vi "SwissSPAD Live_Process Displayed Image.vi"(8 "Error In":errorcluster, 11 "Refnum in":T1) -> (0 "Error Out":errorcluster, 3 "Refnum out":T1)   [LabVIEW 2021]
uses:
  <vilib>/vision/Image Controls.llb/IMAQ Image.ctl
  SwissSPAD Live_Settings List.ctl
  SwissSPAD Live_Image Display Options.ctl
  SwissSPAD Live_Internal Data List.ctl
  Variant/Variant to Data/Variant to Data.lvlib
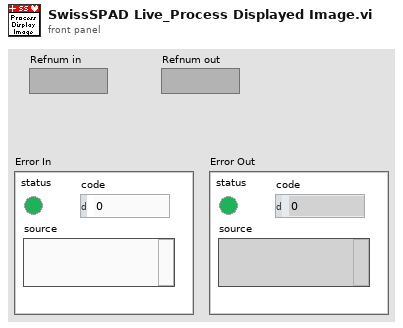
[diagram p1: front panel]
types:
  T1 = typedef "IMAQ Image.ctl" = refnum<image>
  T2 = typedef "SwissSPAD Live_Internal Data List.ctl" = enum16{"Number of pending file saving tasks", "File Saving Tasks Information", "Current Image ROI Information", "# FPGA Reset Attempts", "Histogram Cursor Locations", "Histogram Window is Open"}
  T3 = typedef "SwissSPAD Live_Settings List.ctl" = enum16{"FPGA:Bottom Half", "FPGA:Top Half", "FPGA:Bottom Bitfile Path", "FPGA:Top Bitfile Path", "FPGA:Bottom Bitstream Version", "FPGA:Top Bitstream Version", "FPGA:Auto Reset FPGA", "FPGA:Bottom FPGA Serial Number", "FPGA:Top FPGA Serial Number", "FPGA:Detector PCB Version", "Acquisition Parameters:Microlens", "Acquisition Parameters:SS2 DAQ Parameters", "Acquisition Parameters:Gate Configuration Array", "Acquisition Parameters:SS3 DAQ Parameters", "Acquisition Parameters:Buffer Size (# 8-bit Gates)", "File Information:File Information", "File Information:# Datasets in Series", "File Information:Scrambled File Flag", "File Information:SS3 Gate Slip Correction", "File Information:SS3 Hot Pixel Mismatch Detection", "File Information:Delay between Datasets", "File Information:Save Sum of All Gates Preview", "Image Parameters:Image ROI Information", "Image Parameters:Image Binning Options", "Image Parameters:SS3 Displayed Image", "Image Parameters:Image Display Options", "Image Parameters:Use Histogram Cursors", "Image Parameter:FPGA Data to Display", "UI Settings:Histogram Bins Number", "UI Settings:Histogram Bin Size", "UI Settings:Use Image Display Options", "UI Settings:Verbose Settings", "UI Settings:Verbose Saving"}
  T4 = typedef "SwissSPAD Live_Image Display Options.ctl" = cluster{"Remove Screamers":bool, "Delta":sgl, "Equalize Histogram":bool, "Percentile":sgl, "Hot Pixel Mask Image":path, "Use Hot Pixel Mask":bool}
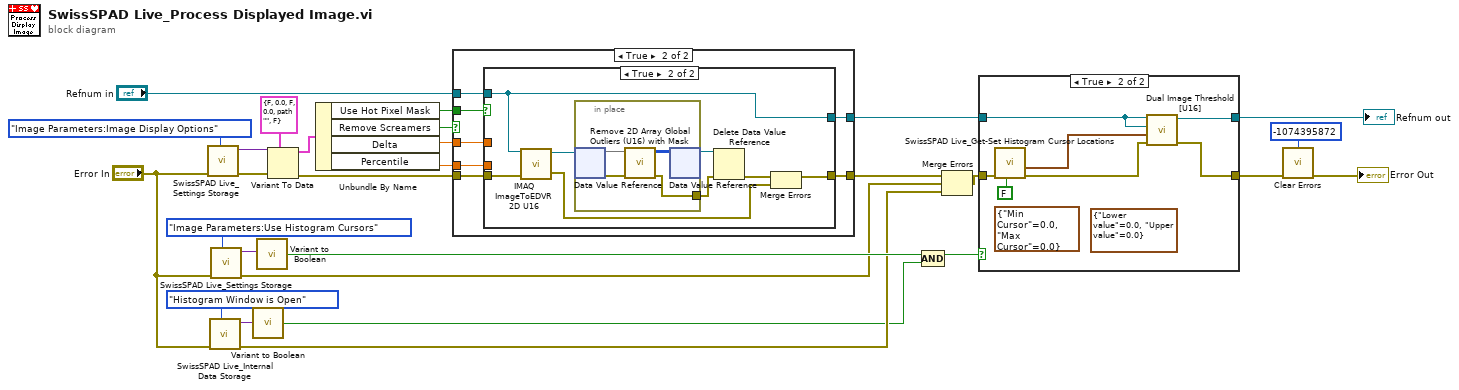
[diagram p0: block diagram]
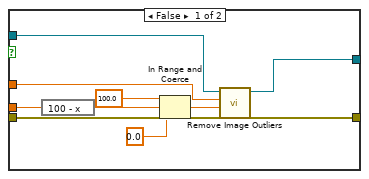
[diagram p4: hidden frame]
diagram:
  n1 = call "SwissSPAD Live_Settings Storage.vi"("Settings List"=SwissSPAD_Live_Settings_List."Image Parameters:Image Display Options", "Error In"="Error In") -> ("Error Out"=w28:errorcluster, "Variant Data out"=w10:variant)  [unwired: 8 in]
  n2 = call "SwissSPAD Live_Internal Data Storage.vi"("SS2 Live Data"=SwissSPAD_Live_Internal_Data_List."Histogram Window is Open", "Error In"="Error In") -> ("Error Out"=w4:errorcluster, "Variant"=w3:variant)  [unwired: 7 in, 1 out]
  n3 = call "SwissSPAD Live_Settings Storage.vi"("Settings List"=SwissSPAD_Live_Settings_List."Image Parameters:Use Histogram Cursors", "Error In"="Error In") -> ("Error Out"=w5:errorcluster, "Variant Data out"=w11:variant)  [unwired: 8 in]
  n4 = call "Variant to Boolean.vi"("Variant"=w3) -> ("Value"=w1:bool)  [unwired: 8 in]
  n5 = call "Variant to Boolean.vi"("Variant"=w11) -> ("Value"=w18:bool)  [unwired: 8 in]
  n6 = Variant To Data(error in=w28, type=T4 {"Remove Screamers"=FALSE, "Delta"=0.0, "Equalize Histogram"=FALSE, "Percentile"=0.0, "Hot Pixel Mask Image"=path "", "Use Hot Pixel Mask"=FALSE} ("Image Display Options"), Variant=w10) -> (data=w26:T4, error out=w25:errorcluster)
  n7 = Unbundle By Name(w26) -> ("Use Hot Pixel Mask"=w9:bool, "Remove Screamers"=w23:bool, "Delta"=w24:sgl, "Percentile"=w21:sgl)
  n8 = case shown="True" w23 {
    tunnel: w25 -> [w29 w37]
    tunnel: w24 -> [_ w36]
    tunnel: [w29 w35] -> w17
    tunnel: "Refnum in" -> [w30 w34]
    tunnel: [w30 w33] -> w16
    tunnel: w21 -> [_ w32]
    tunnel: w9 -> [_ w31]
    frame False {
    }
    frame True {
      n9 = case shown="True" w31 {
        tunnel: w37 -> [w47 w55]
        tunnel: w36 -> [w46 _]
        tunnel: [w45 w49] -> w35
        tunnel: w34 -> [w44 w50]
        tunnel: [w43 w50] -> w33
        tunnel: w32 -> [w42 _]
        frame False {
          n10 = expression code="100 - x"(w42) -> (w41:sgl)
          n11 = In Range and Coerce(upper limit=sgl 100.0, x=w41, lower limit=sgl 0.0) -> (coerced(x)=w40:sgl)  [unwired: 1 out]
          n12 = call "Remove Image Outliers.vi"("error in (no error)"=w47, "Percentile (0-100, Default: ignore)"=w40, "Delta (Default: ignore)"=w46, "Refnum in"=w44) -> ("error out"=w45:errorcluster, "Refnum out"=w43:T1)  [unwired: 6 in]
        }
        frame True {
          n13 = call <vilib>:"IMAQ ImageToEDVR 2D U16.vi"("error out"=w55, "Image"=w50) -> ("error out"=w48:errorcluster, "EDVR 2D U16"=w54:refnum<data-value>)  [unwired: 7 in, 1 out]
          n14 = in-place {
            in-place-border: [w56] -> w52
            n15 = in-place-dvr #1(w54) -> (w59:u16[][], w58:errorcluster)
            n16 = call "Remove 2D Array Global Outliers (U16) with Mask.vi"("Error In"=w58, "2D Array in"=w59) -> ("Error Out"=w56:errorcluster, "2D Array out"=w57:u16[][])  [unwired: 6 in, 2 out]
            n17 = in-place-dvr #1(w57) -> (w53:refnum<data-value>)  [unwired: 1 out]
          }
          n18 = Delete Data Value Reference(data value reference=w53, error in=w52) -> (error out=w51:errorcluster)  [unwired: 1 out]
          n19 = Merge Errors(w51, w48) -> (w49:errorcluster)
        }
      }
    }
  }
  n20 = Compound Arithmetic op=AND(w18, w1) -> (w2:bool)
  n21 = Merge Errors(w17, w5, w4) -> (w6:errorcluster)
  n22 = case shown="True" w2 {
    tunnel: w6 -> [w60 w68]
    tunnel: w16 -> [w61 w62]
    tunnel: [w61 w65] -> w15
    tunnel: [w60 w64] -> w14
    frame False {
    }
    frame True {
      (unwired) cluster{"Lower value":sgl, "Upper value":sgl} {"Lower value"=0.0, "Upper value"=0.0} ("Range")
      (unwired) cluster{"Min Cursor":dbl, "Max Cursor":dbl} {"Min Cursor"=0.0, "Max Cursor"=0.0} ("Histogram Cursor Locations")
      n23 = call "SwissSPAD Live_Get-Set Histogram Cursor Locations.vi"("Get (F)/Set"=FALSE ("Get/Set"), "Error In"=w68) -> ("Error Out"=w67:errorcluster, "Histogram Cursor Locations"=w66:cluster{"Min Cursor":dbl, "Max Cursor":dbl})  [unwired: 7 in, 1 out]
      n24 = call "Dual Image Threshold [U16].vi"("error in (no error)"=w67, "Range"=w66, "Image Dst"=w62, "Image Src"=w62) -> ("error out"=w64:errorcluster, "Image Dst Out"=w65:T1)  [unwired: 5 in, 1 out]
    }
  }
  "Refnum out" <- w15
  n25 = call <vilib>:"Clear Errors.vi"("error in (no error)"=w14, "specific error code to clear (0: all)"=-1074395872) -> ("error out"=→"Error Out":errorcluster)  [unwired: 4 in, 1 out]
